vi "DHE_DRV_get_gain_speed.vi"(0 "fd":i32, 11 "error in (no error)":errorcluster) -> (4 "fd out":i32, 6 "gain":i32, 8 "return value":i32, 10 "speed":i32, 15 "error out":errorcluster)   [LabVIEW 2016]
doc: "This VI closes the I/O interface with the instrument."
uses:
  c/lib/libarcDHE.so
panel:
  in  "s":i32
  in  "g":i32
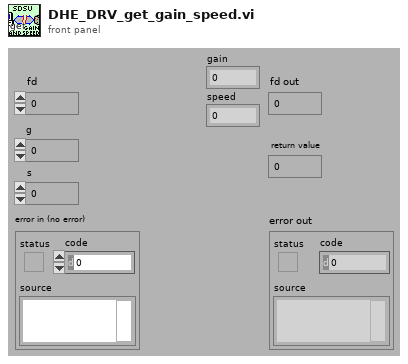
[diagram p1: front panel]
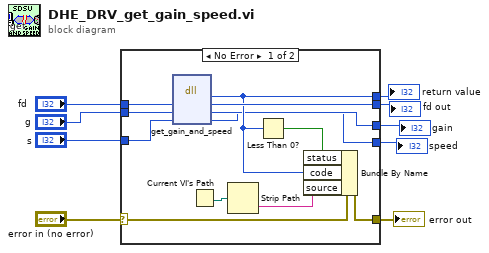
[diagram p0: block diagram]
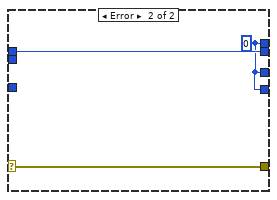
[diagram p2: hidden frame]
diagram:
  n1 = case shown="No Error" "error in (no error)" {
    selector: "error in (no error)" -> [w13 w23]
    tunnel: "fd" -> [w21 w24]
    tunnel: [w12 w22] -> w8
    tunnel: [w17 w23] -> w7
    tunnel: "g" -> [w16 _]
    tunnel: "s" -> [w15 _]
    tunnel: [w14 w24] -> w4
    tunnel: [w11 w22] -> w2
    tunnel: [w10 w22] -> w1
    frame No Error {
      n2 = dll-call lib="home/simager/panview/PAN/Modules/SDSU/private/c/lib/libarcDHE.so" fn="get_gain_and_speed"("fd"=w21, "gain"=w16, "speed"=w15) -> ("return type"=w12:i32, "fd"=w14:i32, "gain"=w11:i32, "speed"=w10:i32)  [unwired: 3 in, 2 out]
      n3 = Current VI's Path() -> (path=w19:path)
      n4 = Strip Path(path=w19) -> (name=w18:string)  [unwired: 1 out]
      n5 = Less Than 0?(x=w12) -> (x < 0?=w20:bool)
      n6 = Bundle By Name(cluster=w13, "status"=w20, "code"=w12, "source"=w18) -> (w17:errorcluster)
    }
    frame Error {
      w22 = 0
    }
  }
  "error out" <- w7
  "return value" <- w8
  "fd out" <- w4
  "gain" <- w2
  "speed" <- w1
